vi "Read Single element from XL.vi"(8 "error in":errorcluster, 9 "Write/Read Cell":T1={"Cell Range"="", "Data 2D"=[], "Select Sheet"="", "1 Data"="", "Data 1D"=[], "Font col"=0, "Bold"=TRUE, "Font Size"=18, "Inside lines"=FALSE}, 10 "Work Sheet":refnum<k7>) -> (0 "error out":errorcluster, 1 "data From XL":string, 2 "Work Sheet":refnum<k7>)   [LabVIEW 2017]
uses:
  controls/read.write.ctl
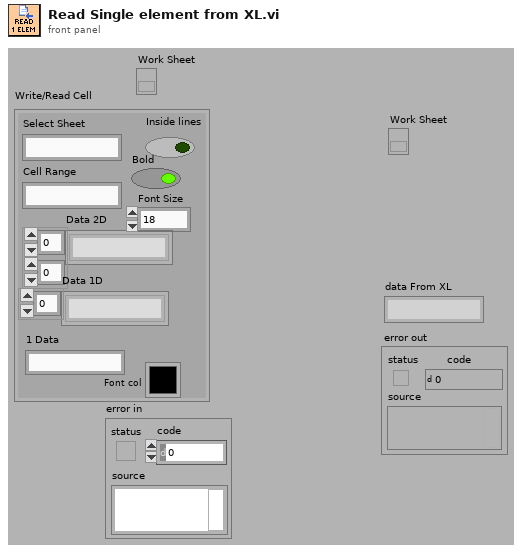
[diagram p1: front panel]
types:
  T1 = typedef "read.write.ctl" = cluster{"Cell Range":string, "Data 2D":string[][], "Select Sheet":string, "1 Data":string, "Data 1D":string[], "Font col":u32, "Bold":bool, "Font Size":i32, "Inside lines":bool}
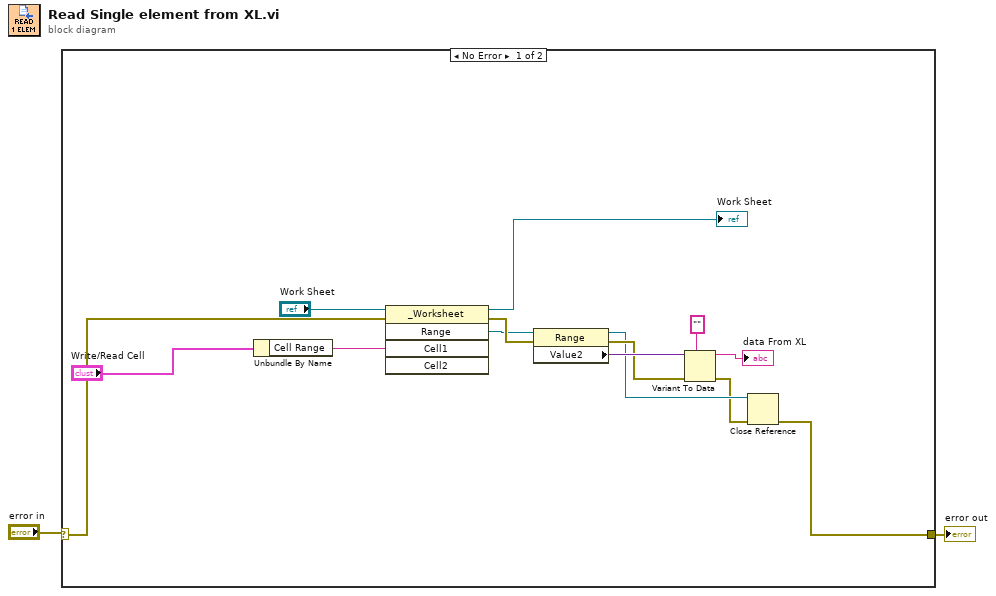
[diagram p0: block diagram]
diagram:
  n1 = case shown="No Error" "error in" {
    selector: "error in" -> [w15 w17]
    tunnel: [w4 w17] -> w1
    frame No Error {
      n2 = Unbundle By Name("Write/Read Cell") -> ("Cell Range"=w8:string)
      n3 = invoke class="_Worksheet" method="Range"(reference="Work Sheet", error in=w15, "Cell1"=w8) -> (reference out=→"Work Sheet":refnum<k7>, error out=w14:errorcluster, "Range"=w11:refnum<k7>)  [unwired: 2 in, 2 out]
      n4 = property class="Range"(reference=w11, error in=w14) -> (reference out=w6:refnum<k7>, error out=w13:errorcluster, "Value2"=w16:variant)
      n5 = Variant To Data(error in=w13, type="", Variant=w16) -> (data=→"data From XL":string, error out=w5:errorcluster)
      n6 = Close Reference(reference=w6, error in (no error)=w5) -> (error out=w4:errorcluster)
    }
    frame Error {
    }
  }
  "error out" <- w1
